vi "GetOrCreateStreamId.vi"(8 "error in (no error)":errorcluster, 9 "operating state":string, 10 "data group":string, 11 "stream Ids":variant) -> (0 "error out":errorcluster, 1 "new streamId":bool, 2 "stream id":string, 3 "streamIds out":variant)   [LabVIEW 2017, in "DataEventCreator.lvlib"]
uses:
  <vilib>/addons/InsightCM/Devices/Shared/Common/DataEventCreator/DataEventCreator.lvlib
  <vilib>/addons/InsightCM/SRP/SRP.lvlib
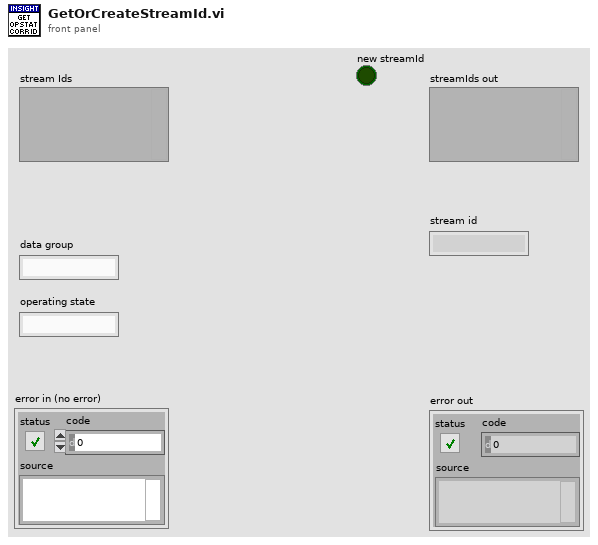
[diagram p1: front panel]
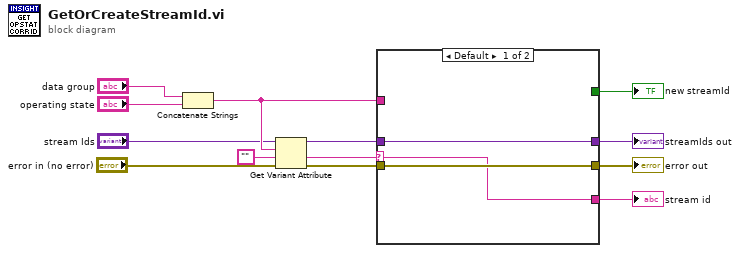
[diagram p0: block diagram]
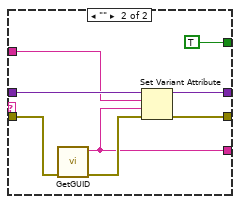
[diagram p2: hidden frame]
diagram:
  n1 = Concatenate Strings("data group", "operating state") -> (w7:string)
  n2 = Get Variant Attribute(Variant="stream Ids", name=w7, default value (empty Variant)="", error in="error in (no error)") -> (duplicate Variant=w5:variant, value=w4:string, error out=w2:errorcluster)  [unwired: 1 out]
  n3 = case shown="Default" w4 {
    selector: w4 -> [w14 _]
    tunnel: w5 -> [w16 w24]
    tunnel: w2 -> [w15 w20]
    tunnel: [w15 w23] -> w11
    tunnel: [w16 w22] -> w10
    tunnel: w7 -> [_ w21]
    tunnel: [w14 w18] -> w9
    tunnel: [_ TRUE] -> w1
    frame Default {
    }
    frame "" {
      n4 = call <vilib>:"GetGUID.vi"("error in (no error)"=w20) -> ("error out"=w19:errorcluster, "GUID"=w18:string)  [unwired: 9 in]
      n5 = Set Variant Attribute(Variant=w24, name=w21, value=w18, error in=w19) -> (Variant out=w22:variant, error out=w23:errorcluster)  [unwired: 1 out]
    }
  }
  "streamIds out" <- w10
  "error out" <- w11
  "stream id" <- w9
  "new streamId" <- w1
